vi "waypoints.vi"(3 "picupLocations":bool[](array[boolean])=[TRUE, TRUE, TRUE], 4 "roadBlocks":bool[][](array[boolean])=[[FALSE, TRUE, FALSE, TRUE, FALSE, FALSE, FALSE], [FALSE, TRUE, FALSE, TRUE, TRUE, TRUE, FALSE], [FALSE, FALSE, FALSE, TRUE, FALSE, FALSE, FALSE], [FALSE, TRUE, FALSE, TRUE, FALSE, TRUE, FALSE], [FALSE, FALSE, FALSE, FALSE, FALSE, FALSE, FALSE]]) -> (1 "waypoints":cluster{"y":dbl, "x":dbl, "stop?":bool}[](array[cluster])=[{"y"=1650.0, "x"=300.0, "stop?"=TRUE}, {"y"=2400.0, "x"=300.0, "stop?"=TRUE}, {"y"=3150.0, "x"=300.0, "stop?"=TRUE}, {"y"=3600.0, "x"=500.0, "stop?"=FALSE}, {"y"=3700.0, "x"=1000.0, "stop?"=FALSE}, {"y"=3700.0, "x"=1390.0, "stop?"=FALSE}, {"y"=2600.0, "x"=1390.0, "stop?"=FALSE}, {"y"=2600.0, "x"=2490.0, "stop?"=FALSE}, {"y"=1500.0, "x"=2490.0, "stop?"=FALSE}, {"y"=1500.0, "x"=3590.0, "stop?"=FALSE}, {"y"=2600.0, "x"=3590.0, "stop?"=FALSE}, {"y"=2600.0, "x"=4690.0, "stop?"=FALSE}, {"y"=3700.0, "x"=4690.0, "stop?"=FALSE}, {"y"=3700.0, "x"=5000.0, "stop?"=FALSE}, {"y"=3600.0, "x"=5500.0, "stop?"=FALSE}, {"y"=2350.0, "x"=5750.0, "stop?"=TRUE}, {"y"=1450.0, "x"=5500.0, "stop?"=FALSE}, {"y"=300.0, "x"=5200.0, "stop?"=FALSE}, {"y"=300.0, "x"=4000.0, "stop?"=FALSE}, {"y"=300.0, "x"=2500.0, "stop?"=FALSE}, {"y"=300.0, "x"=1390.0, "stop?"=FALSE}, {"y"=1500.0, "x"=1390.0, "stop?"=FALSE}, {"y"=2600.0, "x"=1390.0, "stop?"=FALSE}, {"y"=3700.0, "x"=1390.0, "stop?"=FALSE}, {"y"=3700.0, "x"=1000.0, "stop?"=FALSE}, {"y"=3600.0, "x"=500.0, "stop?"=FALSE}, {"y"=1500.0, "x"=500.0, "stop?"=FALSE}, {"y"=250.0, "x"=250.0, "stop?"=TRUE}])   [LabVIEW 2016]
panel:
  in  "return home":cluster{"y":dbl, "x":dbl, "stop?":bool}[](array[cluster])=[{"y"=3700.0, "x"=1000.0, "stop?"=FALSE}, {"y"=3600.0, "x"=500.0, "stop?"=FALSE}, {"y"=1500.0, "x"=500.0, "stop?"=FALSE}, {"y"=250.0, "x"=250.0, "stop?"=FALSE}]
  in  "highway":cluster{"y":dbl, "x":dbl, "stop?":bool}[](array[cluster])=[{"y"=1450.0, "x"=5500.0, "stop?"=FALSE}, {"y"=300.0, "x"=5200.0, "stop?"=FALSE}, {"y"=300.0, "x"=4000.0, "stop?"=FALSE}, {"y"=300.0, "x"=2500.0, "stop?"=FALSE}, {"y"=300.0, "x"=1390.0, "stop?"=FALSE}]
  in  "dropoff section":cluster{"y":dbl, "x":dbl, "stop?":bool}[](array[cluster])=[{"y"=3700.0, "x"=5000.0, "stop?"=FALSE}, {"y"=3600.0, "x"=5500.0, "stop?"=FALSE}, {"y"=2350.0, "x"=5750.0, "stop?"=TRUE}]
  out "Field Map":cluster{dbl[], dbl[]}(graph)={[300.0, 300.0, 300.0, 500.0, 1000.0, 1390.0, 1390.0, 2490.0, 2490.0, 3590.0, 3590.0, 4690.0, 4690.0, 5000.0, 5500.0, 5750.0, 5500.0, 5200.0, 4000.0, 2500.0, 1390.0, 1390.0, 1390.0, 1390.0, 1000.0, 500.0, 500.0, 250.0], [1650.0, 2400.0, 3150.0, 3600.0, 3700.0, 3700.0, 2600.0, 2600.0, 1500.0, 1500.0, 2600.0, 2600.0, 3700.0, 3700.0, 3600.0, 2350.0, 1450.0, 300.0, 300.0, 300.0, 300.0, 1500.0, 2600.0, 3700.0, 3700.0, 3600.0, 1500.0, 250.0]}
  in  "start section":cluster{"y":dbl, "x":dbl, "stop?":bool}[](array[cluster])=[{"y"=1650.0, "x"=300.0, "stop?"=TRUE}, {"y"=2400.0, "x"=300.0, "stop?"=TRUE}, {"y"=3150.0, "x"=300.0, "stop?"=TRUE}, {"y"=3600.0, "x"=500.0, "stop?"=FALSE}, {"y"=3700.0, "x"=1000.0, "stop?"=FALSE}]
  in  "input cluster":cluster{"x":dbl, "y":dbl, "stop?":bool}
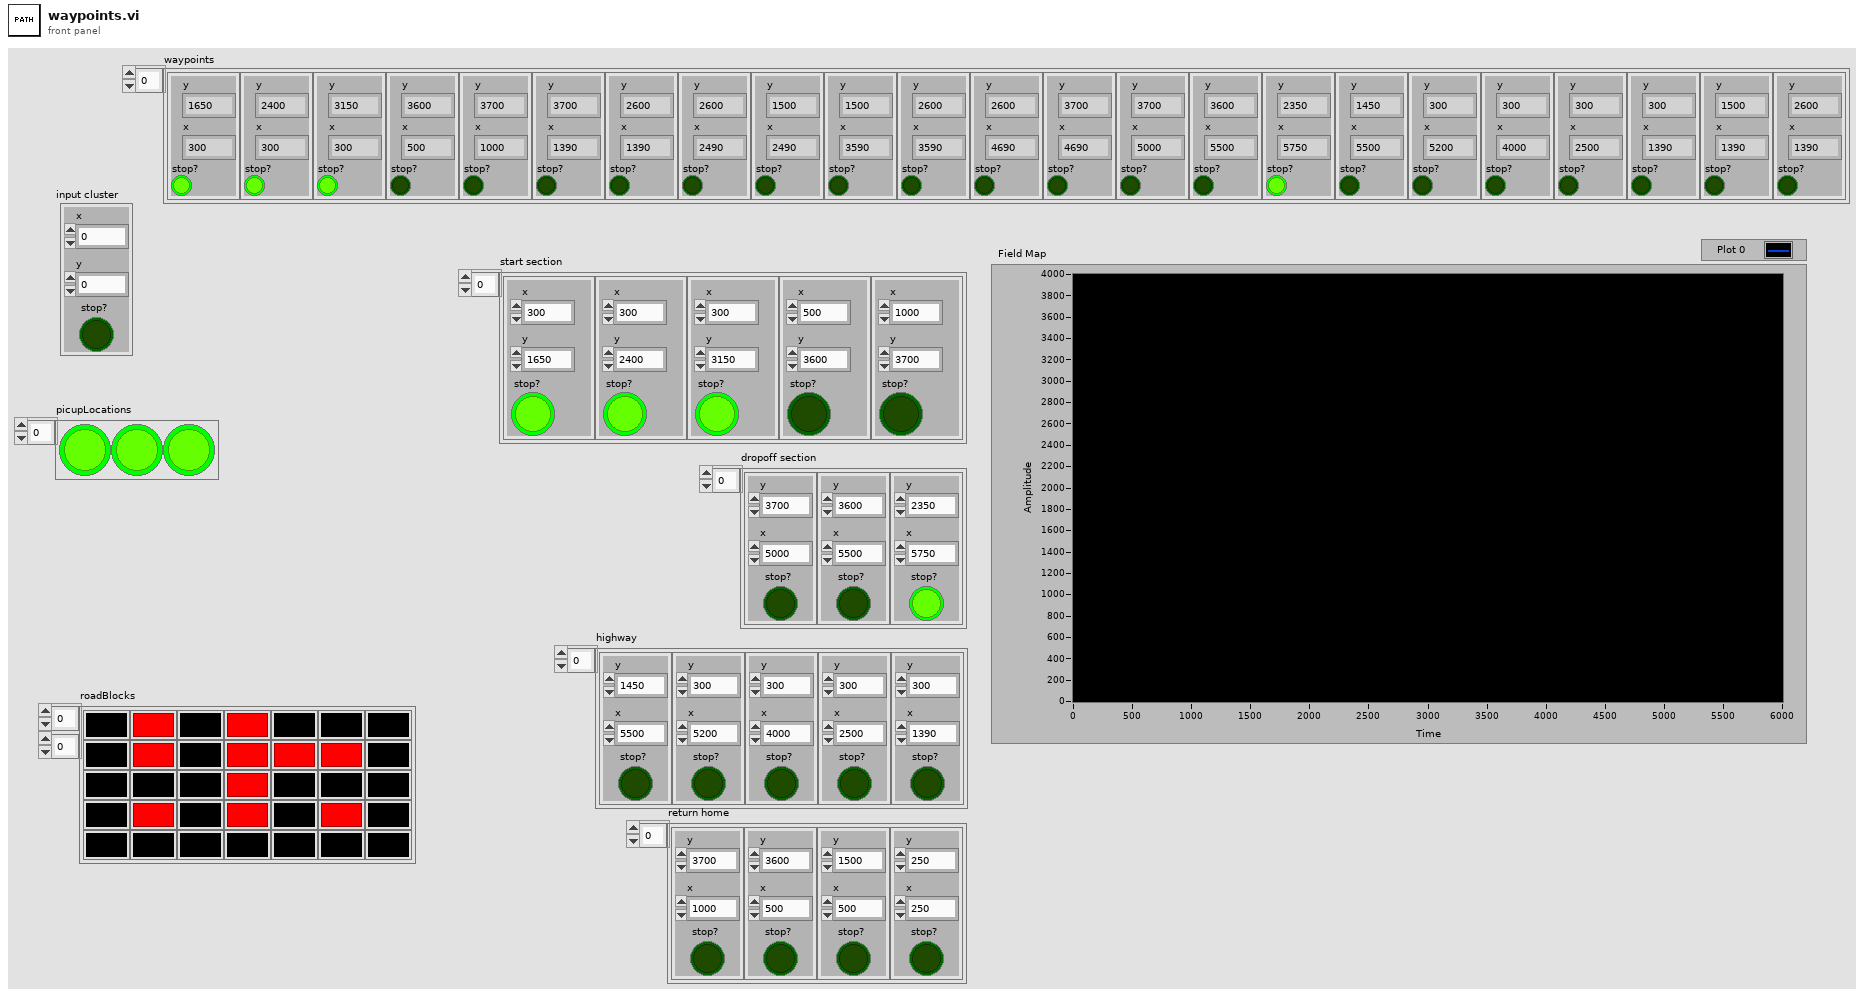
[diagram p1: front panel]
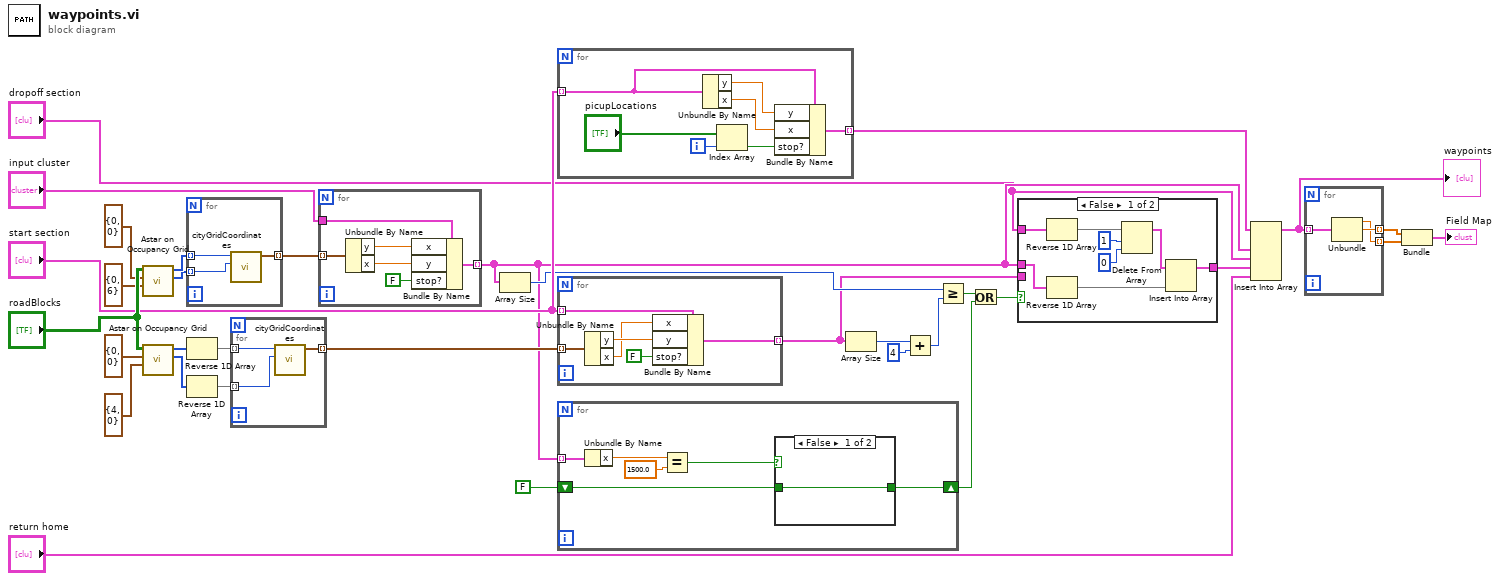
[diagram p0: block diagram]
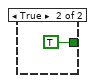
[diagram p2: hidden frame]
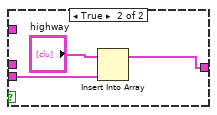
[diagram p3: hidden frame]
diagram:
  n1 = call "Astar on Occupancy Grid.vi"("goal node"=cluster{"X":i32, "Y":i32} {"X"=0, "Y"=6}, "start node"=cluster{"X":i32, "Y":i32} {"X"=0, "Y"=0}, "roadBlocks"="roadBlocks") -> ("y"=w31:i32[], "x"=w32:i32[])  [unwired: 4 in, 1 out]
  n2 = call "Astar on Occupancy Grid.vi"("goal node"=cluster{"X":i32, "Y":i32} {"X"=4, "Y"=0}, "start node"=cluster{"X":i32, "Y":i32} {"X"=0, "Y"=0}, "roadBlocks"="roadBlocks") -> ("y"=w18:i32[], "x"=w17:i32[])  [unwired: 4 in, 1 out]
  n3 = for {
    tunnel: [w36] -> w33 mode=indexing
    tunnel: w32 -> [w35] mode=indexing
    tunnel: w31 -> [w34] mode=indexing
    n4 = call "cityGridCoordinates.vi"("Row"=w34, "Column"=w35) -> ("Cluster"=w36:cluster{"x":dbl, "y":dbl})  [unwired: 9 in]
  }
  n5 = Reverse 1D Array(array=w17) -> (reversed array=w16:i32[])
  n6 = Reverse 1D Array(array=w18) -> (reversed array=w15:i32[])
  n7 = for {
    tunnel: [w39] -> w20 mode=indexing
    tunnel: w16 -> [w38] mode=indexing
    tunnel: w15 -> [w37] mode=indexing
    n8 = call "cityGridCoordinates.vi"("Row"=w37, "Column"=w38) -> ("Cluster"=w39:cluster{"x":dbl, "y":dbl})  [unwired: 9 in]
  }
  n9 = for {
    tunnel: w33 -> [w45] mode=indexing
    tunnel: [w44] -> w9 mode=indexing
    tunnel: "input cluster" -> [w40]
    n10 = Unbundle By Name(w45) -> ("y"=w41:dbl, "x"=w42:dbl)
    n11 = Bundle By Name(cluster=w40, "x"=w41, "y"=w42, "stop?"=FALSE) -> (w44:cluster{"x":dbl, "y":dbl, "stop?":bool})
  }
  n12 = Array Size(array=w9) -> (size(s)=w14:i32)
  n13 = for {
    tunnel: "start section" -> [w52] mode=indexing
    tunnel: [w49] -> w30 mode=indexing
    i -> [w46]
    n14 = Unbundle By Name(w52) -> ("y"=w51:dbl, "x"=w50:dbl)
    n15 = Index Array(array="picupLocations", index=w46) -> (element=w47:bool)
    n16 = Bundle By Name(cluster=w52, "y"=w51, "x"=w50, "stop?"=w47) -> (w49:cluster{"y":dbl, "x":dbl, "stop?":bool})
  }
  n17 = for {
    tunnel: w20 -> [w58] mode=indexing
    tunnel: [w57] -> w10 mode=indexing
    tunnel: "start section" -> [w55] mode=indexing
    n18 = Unbundle By Name(w58) -> ("y"=w54:dbl, "x"=w53:dbl)
    n19 = Bundle By Name(cluster=w55, "x"=w53, "y"=w54, "stop?"=FALSE) -> (w57:cluster{"y":dbl, "x":dbl, "stop?":bool})
  }
  n20 = for {
    tunnel: w9 -> [w64] mode=indexing
    shift-right: [w60] -> w6
    shift-left: FALSE -> [w59]
    n21 = Unbundle By Name(w64) -> ("x"=w63:dbl)
    n22 = Equal?(x=w63, y=1500.0) -> (x = y?=w61:bool)
    n23 = case shown="False" w61 {
      tunnel: [w65 TRUE] -> w60
      tunnel: w59 -> [w65 _]
      frame False {
      }
      frame True {
      }
    }
  }
  n24 = Array Size(array=w10) -> (size(s)=w13:i32)
  n25 = Add(x=w13, y=4) -> (x+y=w12:i32)
  n26 = Greater Or Equal?(x=w14, y=w12) -> (x >= y?=w7:bool)
  n27 = Or(x=w7, y=w6) -> (x .or. y?=w5:bool)
  n28 = case shown="False" w5 {
    tunnel: w9 -> [w73 _]
    tunnel: w10 -> [_ w76]
    tunnel: [w71 w77] -> w3
    tunnel: "dropoff section" -> [w74 _]
    frame False {
      n29 = Reverse 1D Array(array=w74) -> (reversed array=w70:cluster{"y":dbl, "x":dbl, "stop?":bool}[])
      n30 = Reverse 1D Array(array=w73) -> (reversed array=w72:cluster{"x":dbl, "y":dbl, "stop?":bool}[])
      n31 = Delete From Array(array=w70, length=1, index=0) -> (array with subset deleted=w69:cluster{"y":dbl, "x":dbl, "stop?":bool}[])  [unwired: 1 out]
      n32 = Insert Into Array(array=w69, new element=w72) -> (w71:cluster{"y":dbl, "x":dbl, "stop?":bool}[])  [unwired: 1 in]
    }
    frame True {
      n33 = Insert Into Array(array="highway", new element=w76) -> (w77:cluster{"y":dbl, "x":dbl, "stop?":bool}[])  [unwired: 1 in]
    }
  }
  n34 = Insert Into Array(array=w30, new element #1=w9, new element #2="dropoff section", new element #3=w3, new element #4="return home") -> (w4:cluster{"y":dbl, "x":dbl, "stop?":bool}[])  [unwired: 1 in]
  "waypoints" <- w4
  n35 = for {
    tunnel: [w80] -> w29 mode=indexing
    tunnel: [w79] -> w28 mode=indexing
    tunnel: w4 -> [w78] mode=indexing
    n36 = Unbundle(w78) -> ("y"=w79:dbl, "x"=w80:dbl)  [unwired: 1 out]
  }
  n37 = Bundle(w29, w28) -> (→"Field Map":cluster{dbl[], dbl[]})  [unwired: 1 in]
